vi "solar_type Get Bits.vi"(9 "Bit Size (0..64)":i32, 10 "Bit Offset (0)":i32, 11 "Data":string) -> (1 "Value as I32":i32, 2 "Value (Binary) [LVType]":string, 3 "dup Data":string)   [LabVIEW 2018]
doc: "This returns the value from the data string given the bit offset and bit size.\nNote: This handles a bit size no more than 64 bits."
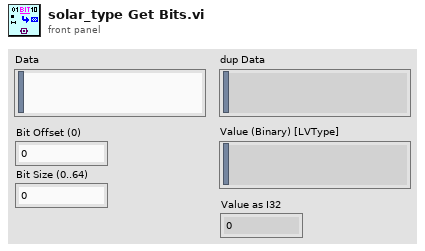
[diagram p1: front panel]
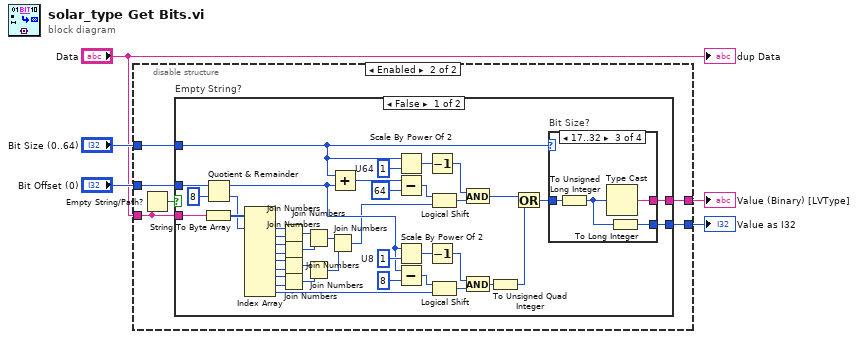
[diagram p0: block diagram]
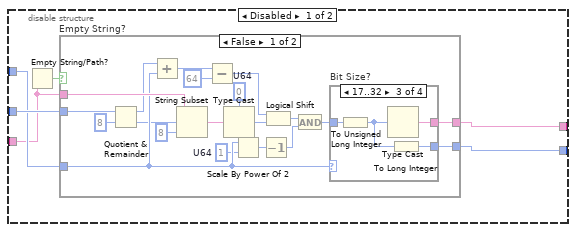
[diagram p2: hidden frame]
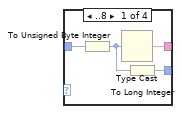
[diagram p3: hidden frame]
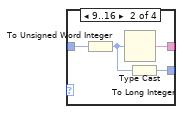
[diagram p4: hidden frame]
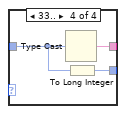
[diagram p5: hidden frame]
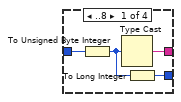
[diagram p7: hidden frame]
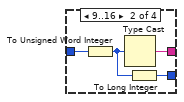
[diagram p8: hidden frame]
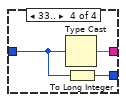
[diagram p9: hidden frame]
diagram:
  n1 = disable-structure shown="Enabled" {
    disable-tunnel: [w11 w52] -> w5
    disable-tunnel: [w9 w50] -> w4
    disable-tunnel: "Bit Offset (0)" -> [w8 w49]
    disable-tunnel: "Bit Size (0..64)" -> [w7 w48]
    disable-tunnel: "Data" -> [w6 w47]
    frame Disabled {
      n2 = Empty String/Path?(string/path=w6) -> (empty?=w10:bool)
      n3 = case "Empty String?" shown="False" w10 {
        tunnel: w6 -> [w31 _]
        tunnel: [w30 _] -> w11
        tunnel: [w29 _] -> w9
        tunnel: w8 -> [w28 _]
        tunnel: w7 -> [w27 _]
        frame False {
          w17 = u64 1  # U64
          w21 = u64 0  # U64
          n4 = Quotient & Remainder(x=w28, y=8) -> (x-y*floor(x/y)=w24:i32, floor(x/y)=w25:i32)
          n5 = Add(x=w24, y=w27) -> (x+y=w22:i32)
          n6 = String Subset(string=w31, offset (0)=w25, length (rest)=8 ("length (rest)")) -> (substring=w23:string)
          n7 = Subtract(x=w22, y=64) -> (x-y=w14:i32)
          n8 = Type Cast(type=w21, x=w23) -> (*(type *) &x=w20:u64)
          n9 = Scale By Power Of 2(n=w27, x=w17) -> (x*2^n=w16:u64)
          n10 = Decrement(x=w16) -> (x-1=w15:u64)
          n11 = Logical Shift(y=w14, x=w20) -> (x << y=w18:u64)
          n12 = And(x=w18, y=w15) -> (x .and. y?=w13:u64)
          n13 = case "Bit Size?" shown="17..32" w27 {
            tunnel: [w35 w39 w43 w46] -> w30
            tunnel: w13 -> [w34 w38 w42 w45]
            tunnel: [w32 w36 w40 w44] -> w29
            frame ..8 {
              n14 = To Unsigned Byte Integer(number=w34) -> (unsigned 8bit integer=w33:u8)
              n15 = Type Cast(x=w33) -> (*(type *) &x=w35:string)  [unwired: 1 in]
              n16 = To Long Integer(number=w33) -> (32bit integer=w32:i32)
            }
            frame 9..16 {
              n17 = To Unsigned Word Integer(number=w38) -> (unsigned 16bit integer=w37:u16)
              n18 = Type Cast(x=w37) -> (*(type *) &x=w39:string)  [unwired: 1 in]
              n19 = To Long Integer(number=w37) -> (32bit integer=w36:i32)
            }
            frame 17..32 {
              n20 = To Unsigned Long Integer(number=w42) -> (unsigned 32bit integer=w41:u32)
              n21 = Type Cast(x=w41) -> (*(type *) &x=w43:string)  [unwired: 1 in]
              n22 = To Long Integer(number=w41) -> (32bit integer=w40:i32)
            }
            frame 33.. {
              n23 = Type Cast(x=w45) -> (*(type *) &x=w46:string)  [unwired: 1 in]
              n24 = To Long Integer(number=w45) -> (32bit integer=w44:i32)
            }
          }
        }
        frame True {
        }
      }
    }
    frame Enabled {
      n25 = Empty String/Path?(string/path=w47) -> (empty?=w51:bool)
      n26 = case "Empty String?" shown="False" w51 {
        tunnel: w47 -> [w82 _]
        tunnel: [w94 _] -> w52
        tunnel: [w93 _] -> w50
        tunnel: w49 -> [w92 _]
        tunnel: w48 -> [w91 _]
        frame False {
          w65 = u8 1  # U8
          w86 = u64 1  # U64
          n27 = String To Byte Array(string=w82) -> (unsigned byte array=w81:u8[])
          n28 = Quotient & Remainder(x=w92, y=8) -> (x-y*floor(x/y)=w64:i32, floor(x/y)=w54:i32)
          n29 = Index Array(array=w81, index #1=w54) -> (element #1=w80:u8, element #2=w79:u8, element #3=w78:u8, element #4=w77:u8, element #5=w76:u8, element #6=w75:u8, element #7=w74:u8, element #8=w73:u8, element #9=w60:u8)  [unwired: 8 in]
          n30 = Join Numbers(hi=w80, lo=w79) -> ((hi.lo)=w72:u16)
          n31 = Join Numbers(hi=w78, lo=w77) -> ((hi.lo)=w70:u16)
          n32 = Join Numbers(hi=w76, lo=w75) -> ((hi.lo)=w71:u16)
          n33 = Join Numbers(hi=w74, lo=w73) -> ((hi.lo)=w69:u16)
          n34 = Join Numbers(hi=w72, lo=w70) -> ((hi.lo)=w68:u32)
          n35 = Join Numbers(hi=w71, lo=w69) -> ((hi.lo)=w67:u32)
          n36 = Join Numbers(hi=w68, lo=w67) -> ((hi.lo)=w53:u64)
          n37 = Add(x=w91, y=w64) -> (x+y=w89:i32)
          n38 = Scale By Power Of 2(n=w91, x=w86) -> (x*2^n=w85:u64)
          n39 = Subtract(x=w89, y=64) -> (x-y=w83:i32)
          n40 = Scale By Power Of 2(n=w64, x=w65) -> (x*2^n=w66:u8)
          n41 = Subtract(x=w64, y=8) -> (x-y=w61:i32)
          n42 = Decrement(x=w85) -> (x-1=w84:u64)
          n43 = Decrement(x=w66) -> (x-1=w62:u8)
          n44 = Logical Shift(y=w83, x=w53) -> (x << y=w87:u64)
          n45 = Logical Shift(y=w61, x=w60) -> (x << y=w59:u8)
          n46 = And(x=w84, y=w87) -> (x .and. y?=w56:u64)
          n47 = And(x=w62, y=w59) -> (x .and. y?=w58:u8)
          n48 = To Unsigned Quad Integer(1:w58) -> (0:w57:u64)
          n49 = Or(x=w56, y=w57) -> (x .or. y?=w55:u64)
          n50 = case "Bit Size?" shown="17..32" w91 {
            tunnel: [w98 w102 w106 w109] -> w94
            tunnel: w55 -> [w97 w101 w105 w108]
            tunnel: [w95 w99 w103 w107] -> w93
            frame ..8 {
              n51 = To Unsigned Byte Integer(number=w97) -> (unsigned 8bit integer=w96:u8)
              n52 = Type Cast(x=w96) -> (*(type *) &x=w98:string)  [unwired: 1 in]
              n53 = To Long Integer(number=w96) -> (32bit integer=w95:i32)
            }
            frame 9..16 {
              n54 = To Unsigned Word Integer(number=w101) -> (unsigned 16bit integer=w100:u16)
              n55 = Type Cast(x=w100) -> (*(type *) &x=w102:string)  [unwired: 1 in]
              n56 = To Long Integer(number=w100) -> (32bit integer=w99:i32)
            }
            frame 17..32 {
              n57 = To Unsigned Long Integer(number=w105) -> (unsigned 32bit integer=w104:u32)
              n58 = Type Cast(x=w104) -> (*(type *) &x=w106:string)  [unwired: 1 in]
              n59 = To Long Integer(number=w104) -> (32bit integer=w103:i32)
            }
            frame 33.. {
              n60 = Type Cast(x=w108) -> (*(type *) &x=w109:string)  [unwired: 1 in]
              n61 = To Long Integer(number=w108) -> (32bit integer=w107:i32)
            }
          }
        }
        frame True {
        }
      }
    }
  }
  "Value (Binary) [LVType]" <- w5
  "Value as I32" <- w4
  "dup Data" <- "Data"
